vi "saveSetup.vi"(6 "Configuration":T4={"Primary Filter"="<NO FILTER>", "Secondary Filter"="<NO FILTER>", "Slit Mask"="<NO MASK>", "Grating"="<NO GRATING>", "CS Target"=0.0, "GS Target"=0.0, "Coll Focus"=1000, "Camera Focus"=0, "Name"="", "User"="", "Date"="", "Comment"="", "use Flexure Comp?"=FALSE, "Select Mode:"=0} {"Select Mode:" items=["Custom", "Imaging", "300 All", "600 UV", "600 Blue", "600 Mid", "600 Red", "1200 m0", "1200 m1", "1200 m2", "1200 m3", "1200 m4", "1200 m5", "1200 m6", "1200 m7", "1200 RESOLVE", "400 m1", "400 m2", "930 m1", "930 m2", "930 m3", "930 m4", "930 m5", "930 m6", "400WD", "930TP", "400Fermi", "400Padgett", "400Lewis", "400Crotts", "600BLee", "600RLee", "400WW"]}) -> (0 "error out":errorcluster, 1 "Canceled?":bool, 2 "Configuration Written":T3 {"Select Mode:" items=["Custom", "Imaging", "300 All", "600 UV", "600 Blue", "600 Mid", "600 Red", "1200 m0", "1200 m1", "1200 m2", "1200 m3", "1200 m4", "1200 m5", "1200 m6", "1200 m7", "1200 RESOLVE", "400 m1", "400 m2", "930 m1", "930 m2", "930 m3", "930 m4", "930 m5", "930 m6", "400KL"]})   [LabVIEW 2015]
uses:
  Utils/GSP_ObsConfig.llb/configuration.ctl
  Users/Stephen/Desktop/BETA_GSCS - Copy/GUI/GSP_GUI_global.vi
panel:
  in  "Master Config Location":path
  out "grating index":dbl
  out "Gratings":T1(array[cluster])
  in  "Littrow Config":dbl
  out "Array":T2(array[cluster])
  in  "Save to":path
  out "Status":string
  in  "Save":bool
  in  "Configuration Name":string="default"
  # "Central Wavelength (mm)"
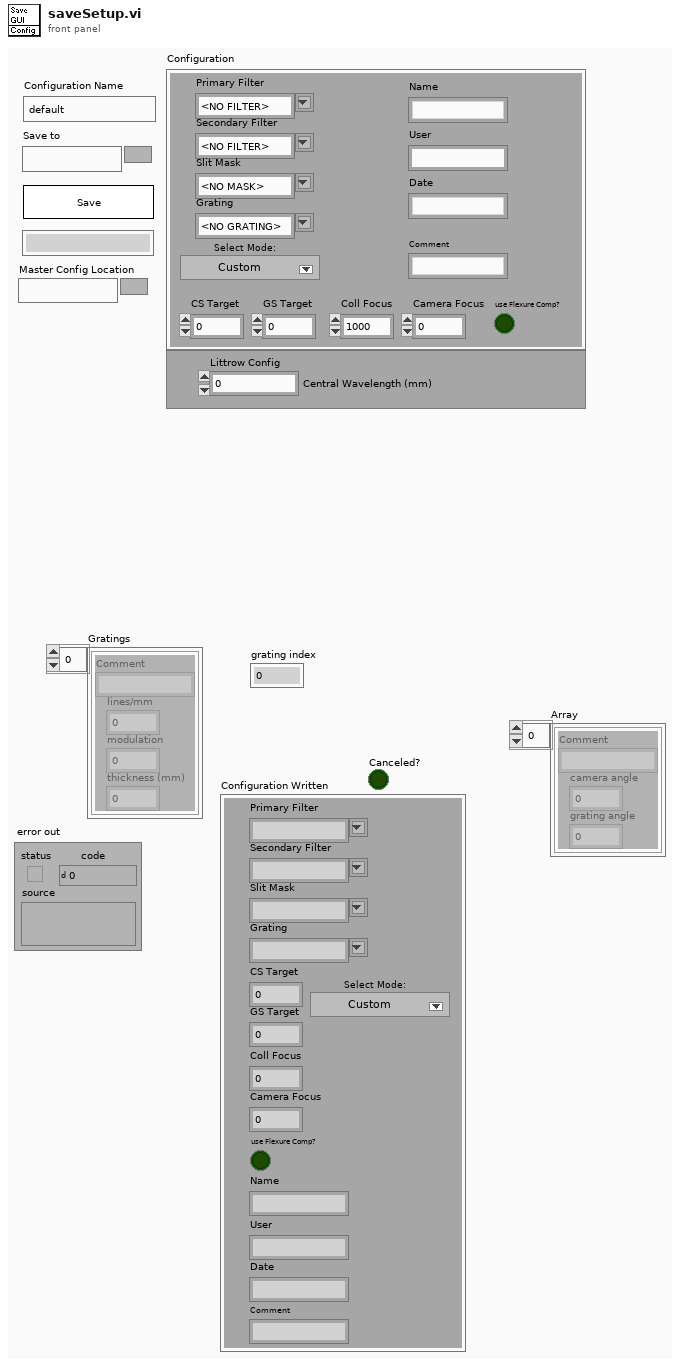
[diagram p1: front panel]
types:
  T1 = cluster{"Comment":string, "lines/mm":i32, "modulation":dbl, "thickness (mm)":dbl}[]
  T2 = cluster{"Comment":string, "camera angle":dbl, "grating angle":dbl}[]
  T3 = typedef "configuration.ctl" = cluster{"Primary Filter":string, "Secondary Filter":string, "Slit Mask":string, "Grating":string, "CS Target":dbl, "GS Target":dbl, "Coll Focus":i32, "Camera Focus":i32, "Name":string, "User":string, "Date":string, "Comment":string, "use Flexure Comp?":bool, "Select Mode:":u16}
  T4 = cluster{"Primary Filter":string, "Secondary Filter":string, "Slit Mask":string, "Grating":string, "CS Target":dbl, "GS Target":dbl, "Coll Focus":i32, "Camera Focus":i32, "Name":string, "User":string, "Date":string, "Comment":string, "use Flexure Comp?":bool, "Select Mode:":u16}
  T5 = cluster{"Comment":string, "lines/mm":i32, "modulation":dbl, "thickness (mm)":dbl}
  T6 = cluster{"Primary Filter Names":string[], "Secondary Filter Names":string[], "Grating Names":string[], "Slit Mask Names":string[], "Standard Observing Modes":string[]}
  T7 = cluster{"Comment":string, "camera angle":dbl, "grating angle":dbl}
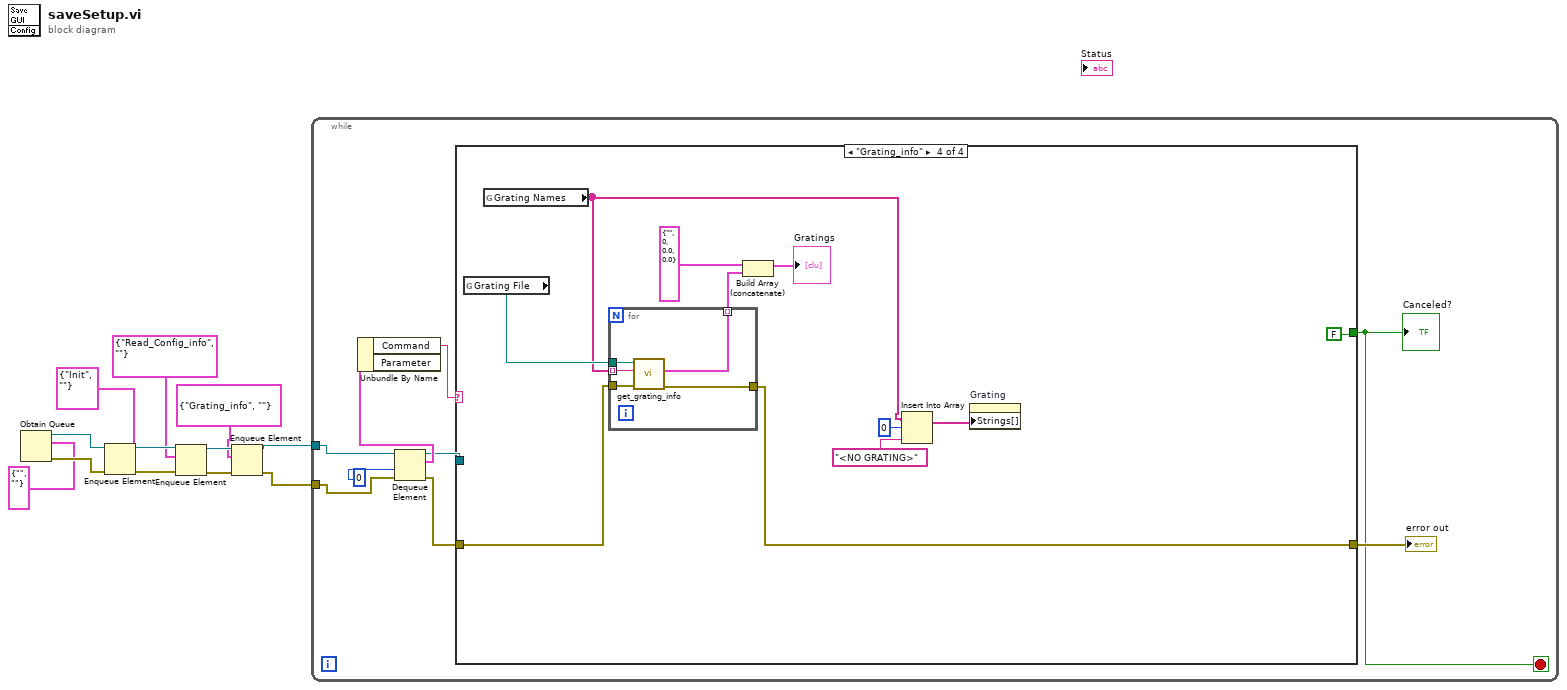
[diagram p0: block diagram]
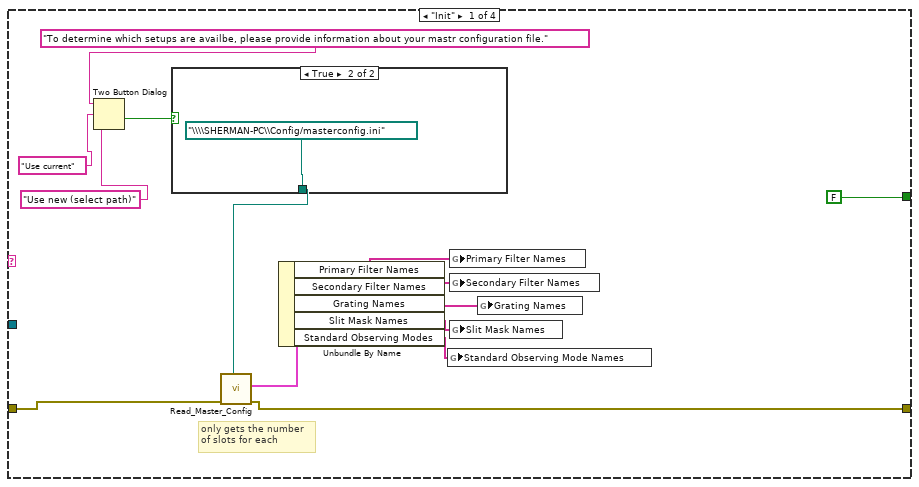
[diagram p2: hidden frame]
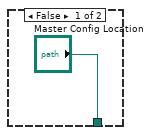
[diagram p3: hidden frame]
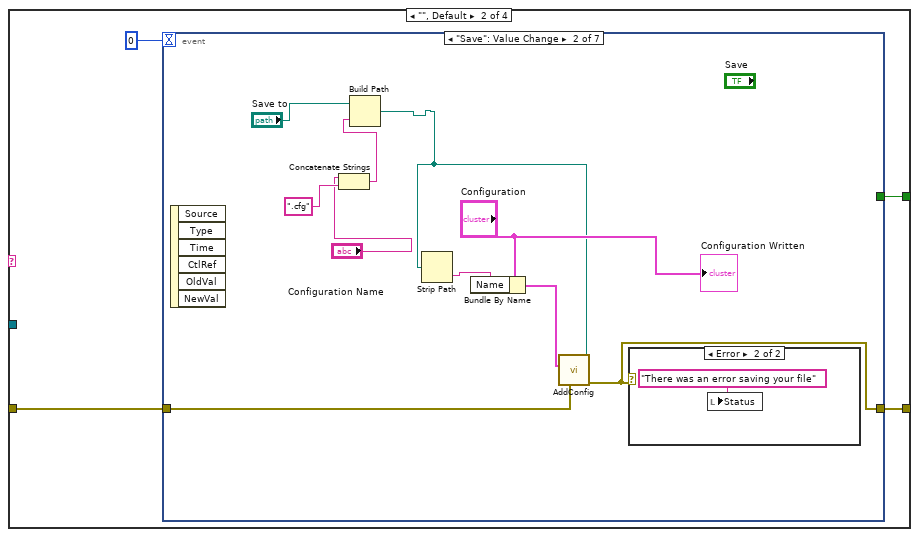
[diagram p4: hidden frame]
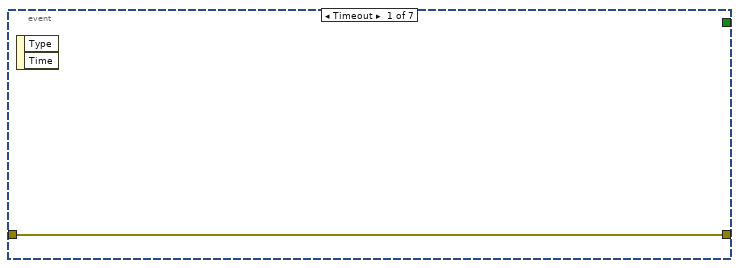
[diagram p5: hidden frame]
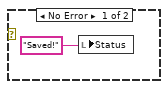
[diagram p6: hidden frame]
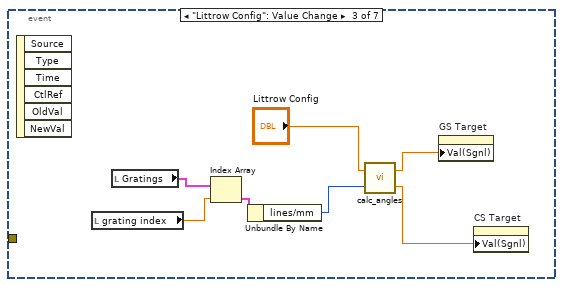
[diagram p7: hidden frame]
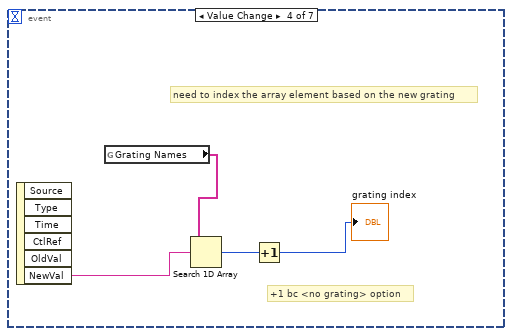
[diagram p8: hidden frame]
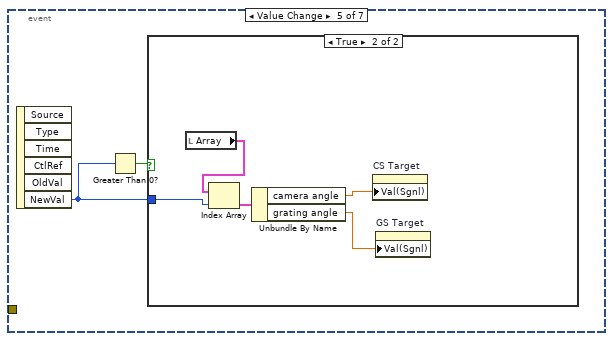
[diagram p9: hidden frame]
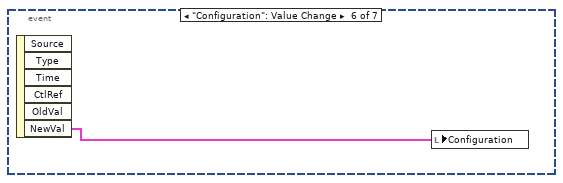
[diagram p11: hidden frame]
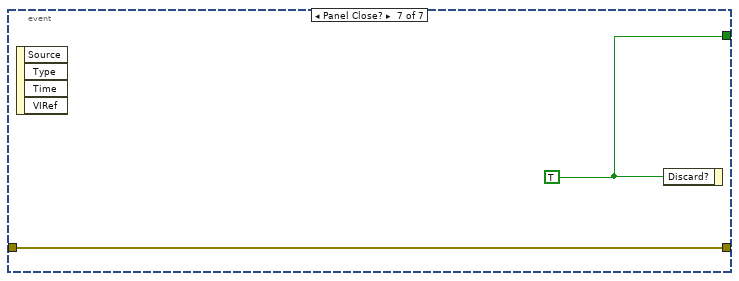
[diagram p12: hidden frame]
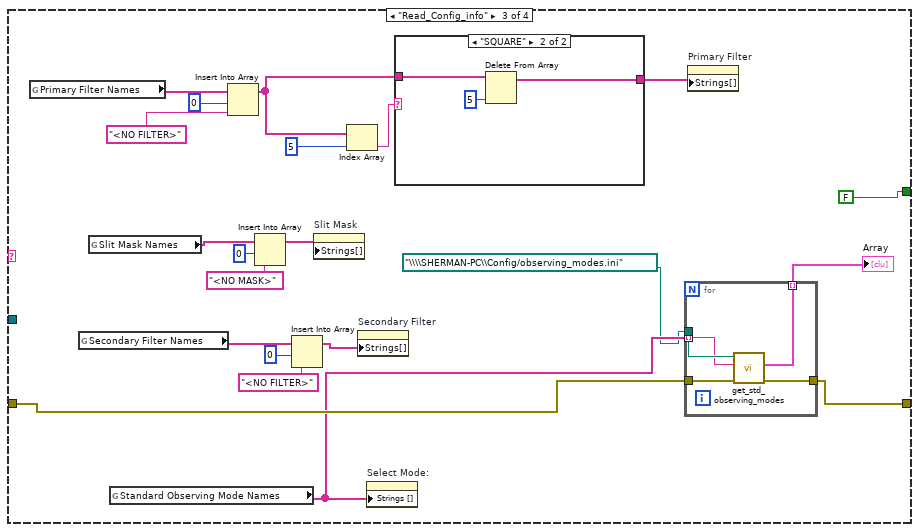
[diagram p13: hidden frame]
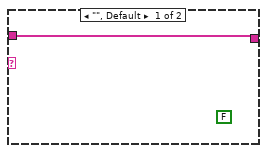
[diagram p14: hidden frame]
diagram:
  n1 = Obtain Queue(element data type=cluster{"\nCommand":string, "Parameter":string} {"\nCommand"="", "Parameter"=""}) -> (queue out=w11:refnum<queue>, error out=w10:errorcluster)  [unwired: 4 in, 1 out]
  n2 = Enqueue Element(queue=w11, element=cluster{string, string} {"Init", ""}, error in (no error)=w10) -> (queue out=w8:refnum<queue>, error out=w7:errorcluster)  [unwired: 1 in, 1 out]
  n3 = Enqueue Element(queue=w8, element=cluster{string, string} {"Read_Config_info", ""}, error in (no error)=w7) -> (queue out=w3:refnum<queue>, error out=w4:errorcluster)  [unwired: 1 in, 1 out]
  n4 = Enqueue Element(queue=w3, element=cluster{string, string} {"Grating_info", ""}, error in (no error)=w4) -> (queue out=w6:refnum<queue>, error out=w5:errorcluster)  [unwired: 1 in, 1 out]
  n5 = while {
    tunnel: w5 -> [w15]
    tunnel: w6 -> [w16]
    stop <- w20 stop-if-true
    n6 = Dequeue Element(queue=w16, timeout in ms (-1)=0, error in (no error)=w15) -> (queue out=w13:refnum<queue>, element=w17:cluster{"\nCommand":string, "Parameter":string}, error out=w14:errorcluster)  [unwired: 1 out]
    n7 = Unbundle By Name(w17) -> ("Command"=w18:string)  [unwired: 1 out]
    n8 = case shown="\"Grating_info\"" w18 {
      tunnel: w14 -> [w29 w41 w79 w108]
      tunnel: [w28 w40 w78 w107] -> w21
      tunnel: [FALSE w39 FALSE FALSE] -> w20
      tunnel: w13 -> [_ _ _ _]
      frame "Init" {
        # "only gets the number\nof slots for each"
        n9 = Two Button Dialog(message="To determine which setups are availbe, please provide information about your mastr configuration file.", 1:"Use new (select path)", 2:"Use current") -> (T button?=w26:bool)
        n10 = case shown="True" w26 {
          tunnel: ["Master Config Location" path "\\\\SHERMAN-PC\\Config/masterconfig.ini"] -> w22
          frame False {
          }
          frame True {
          }
        }
        n11 = call "Read_Master_Config.vi"("error in (no error)"=w29, "configuration file path"=w22) -> ("error out"=w28:errorcluster, "Present Configuration"=w31:T6)  [unwired: 3 in, 1 out]
        n12 = Unbundle By Name(w31) -> ("Primary Filter Names"=w32:string[], "Secondary Filter Names"=w33:string[], "Grating Names"=w34:string[], "Slit Mask Names"=w35:string[], "Standard Observing Modes"=w30:string[])
        n13 = global write "GSP_GUI_global.vi" "Standard Observing Mode Names"(w30) -> ()
        n14 = global write "GSP_GUI_global.vi" "Primary Filter Names"(w32) -> ()
        n15 = global write "GSP_GUI_global.vi" "Secondary Filter Names"(w33) -> ()
        n16 = global write "GSP_GUI_global.vi" "Slit Mask Names"(w35) -> ()
        n17 = global write "GSP_GUI_global.vi" "Grating Names"(w34) -> ()
      }
      frame "", Default {
        n18 = event shown="[1] \"Save\": Value Change" {
          selector: _ -> [_ _ _ _ _ _ _]
          dyn-events: _ -> [_ _ _ _ _ _ _]
          timeout: 0 -> [_ _ _ _ _ _ _]
          tunnel: [_ _ _ _ _ _ w74] -> w39
          tunnel: w41 -> [w42 w52 _ _ _ _ w75]
          tunnel: [w42 w47 _ _ _ _ w75] -> w40
          event Timeout {
            n19 = event-data() -> ()  [unwired: 1 in, 2 out]
          }
          event "Save": Value Change {
            n20 = event-data() -> ()  [unwired: 1 in, 6 out]
            n21 = Concatenate Strings("Configuration Name", ".cfg") -> (w43:string)
            n22 = Build Path(base path="Save to", name or relative path=w43) -> (appended path=w46:path)
            n23 = Strip Path(path=w46) -> (name=w48:string)  [unwired: 1 out]
            n24 = Bundle By Name(cluster="Configuration", "Name"=w48) -> (w51:T4)
            n25 = call "AddConfig.vi"("error in (no error)"=w52, "Configuration In"=w51, "path"=w46) -> ("error out"=w47:errorcluster)  [unwired: 4 in]
            n26 = case shown="Error" w47 {
              frame No Error {
                n27 = local write "Status"("Saved!") -> ()
              }
              frame Error {
                n28 = local write "Status"("There was an error saving your file") -> ()
              }
            }
            "Configuration Written" <- "Configuration"
          }
          event "Littrow Config": Value Change {
            n29 = event-data() -> ()  [unwired: 1 in, 6 out]
            n30 = local read "grating index"() -> (w58:dbl)
            n31 = local read "Gratings"() -> (w57:T1)
            n32 = Index Array(array=w57, index=w58) -> (element=w56:T5)
            n33 = Unbundle By Name(w56) -> ("lines/mm"=w55:i32)
            n34 = call "calc_angles.vi"("lines/mm"=w55, "Central Wavlength (nm)"="Littrow Config") -> ("camera angle"=w60:dbl, "grating angle"=w59:dbl)
            n35 = property on="GS Target" class="DigNum (strict)"("Val(Sgnl)"=w59) -> ()  [unwired: 2 in, 2 out]
            n36 = property on="CS Target" class="DigNum (strict)"("Val(Sgnl)"=w60) -> ()  [unwired: 2 in, 2 out]
          }
          event "Configuration.Grating": Value Change {
            # "+1 bc <no grating> option"
            # "need to index the array element based on the new grating"
            n37 = event-data() -> ("NewVal"=w65:string)  [unwired: 1 in, 5 out]
            n38 = global read "GSP_GUI_global.vi" "Grating Names"() -> (w64:string[])
            n39 = Search 1D Array(1D array=w64, element=w65) -> (index of element=w63:i32)  [unwired: 1 in]
            n40 = Increment(x=w63) -> (x+1=→"grating index":i32)
          }
          event "Configuration.Select Mode:": Value Change {
            n41 = event-data() -> ("NewVal"=w66:u16)  [unwired: 1 in, 5 out]
            n42 = Greater Than 0?(x=w66) -> (x > 0?=w67:bool)
            n43 = case shown="True" w67 {
              tunnel: w66 -> [_ w72]
              frame False {
              }
              frame True {
                n44 = local read "Array"() -> (w71:T2)
                n45 = Index Array(array=w71, index=w72) -> (element=w70:T7)
                n46 = Unbundle By Name(w70) -> ("camera angle"=w69:dbl, "grating angle"=w68:dbl)
                n47 = property on="CS Target" class="DigNum (strict)"("Val(Sgnl)"=w69) -> ()  [unwired: 2 in, 2 out]
                n48 = property on="GS Target" class="DigNum (strict)"("Val(Sgnl)"=w68) -> ()  [unwired: 2 in, 2 out]
              }
            }
          }
          event "Configuration": Value Change {
            n49 = event-data() -> ("NewVal"=w73:T4)  [unwired: 1 in, 5 out]
            n50 = local write "Configuration"(w73) -> ()
          }
          event Panel Close? {
            w74 = TRUE
            n51 = event-data() -> ()  [unwired: 1 in, 4 out]
            n52 = event-data("Discard?"=w74) -> ()  [unwired: 1 in, 1 out]
          }
        }
      }
      frame "Read_Config_info" {
        n53 = global read "GSP_GUI_global.vi" "Primary Filter Names"() -> (w95:string[])
        n54 = global read "GSP_GUI_global.vi" "Secondary Filter Names"() -> (w83:string[])
        n55 = global read "GSP_GUI_global.vi" "Slit Mask Names"() -> (w89:string[])
        n56 = global read "GSP_GUI_global.vi" "Standard Observing Mode Names"() -> (w77:string[])
        n57 = Insert Into Array(array=w95, index=0, new element="<NO FILTER>" ("new element/subarray")) -> (w93:string[])
        n58 = Insert Into Array(array=w89, index=0, new element="<NO MASK>" ("new element/subarray")) -> (w86:string[])
        n59 = Insert Into Array(array=w83, index=0, new element="<NO FILTER>" ("new element/subarray")) -> (w82:string[])
        n60 = property on="Slit Mask" class="CmbBox"("Strings[]"=w86) -> ()  [unwired: 2 in, 2 out]
        n61 = Index Array(array=w93, index=5) -> (element=w91:string)
        n62 = property on="Secondary Filter" class="CmbBox"("Strings[]"=w82) -> ()  [unwired: 2 in, 2 out]
        n63 = property on="Select Mode:" class="Ring (strict)"("Strings []"=w77) -> ()  [unwired: 2 in, 2 out]
        n64 = case shown="\"SQUARE\"" w91 {
          tunnel: w93 -> [w102 w105]
          tunnel: [w102 w103] -> w90
          frame "", Default {
            (unwired) FALSE ("5 hole or 6 hole wheel?")
          }
          frame "SQUARE" {
            n65 = Delete From Array(array=w105, index=5) -> (array with subset deleted=w103:string[])  [unwired: 1 in, 1 out]
          }
        }
        n66 = for {
          tunnel: w77 -> [w100] mode=indexing
          tunnel: path "\\\\SHERMAN-PC\\Config/observing_modes.ini" -> [w101]
          tunnel: w79 -> [w99]
          tunnel: [w98] -> w78
          tunnel: [w97] -> w80 mode=indexing
          n67 = call "get_std_observing_modes.vi"("error in (no error)"=w99, "mode name"=w100, "configuration file path"=w101) -> ("error out"=w98:errorcluster, "Standard Mode Info"=w97:T7)  [unwired: 3 in]
        }
        "Array" <- w80
        n68 = property on="Primary Filter" class="CmbBox"("Strings[]"=w90) -> ()  [unwired: 2 in, 2 out]
      }
      frame "Grating_info" {
        n69 = global read "GSP_GUI_global.vi" "Grating File"() -> (w113:path)
        n70 = global read "GSP_GUI_global.vi" "Grating Names"() -> (w109:string[])
        n71 = for {
          tunnel: [w121] -> w112 mode=indexing
          tunnel: [w120] -> w107
          tunnel: w109 -> [w119] mode=indexing
          tunnel: w113 -> [w118]
          tunnel: w108 -> [w117]
          n72 = call "get_grating_info.vi"("error in (no error)"=w117, "grating name"=w119, "configuration file path"=w118) -> ("error out"=w120:errorcluster, "Grating Info"=w121:T5)  [unwired: 3 in]
        }
        n73 = Build Array (concatenate)(T5 {"Comment"="", "lines/mm"=0, "modulation"=0.0, "thickness (mm)"=0.0} ("Grating Info"), w112) -> (→"Gratings":T1)
        n74 = Insert Into Array(array=w109, index=0, new element="<NO GRATING>" ("new element/subarray")) -> (w114:string[])
        n75 = property on="Grating" class="CmbBox"("Strings[]"=w114) -> ()  [unwired: 2 in, 2 out]
      }
    }
    "error out" <- w21
    "Canceled?" <- w20
  }
